vi "novoGoleiroGoleiroForaDaArea.vi"(9 "Goleiro.Xpadrão":dbl=80.0 format="%#_13g", 10 "Robot in":T1, 11 "IA State":T6={"our_robots"=[], "enemy_robots"=[], "balls"=[], "geometry"={"field_length"=0, "field_width"=0, "goal_width"=0, "goal_depth"=0, "center_circle_radius"=0, "defense_width"=0, "defense_depth"=0, "free_kick_from_defense_dist"=0, "penalty_spot_from_field_line_dist"=0, "penalty_line_from_spot_dist"=0, "half_moon_depth"=0, "half_moon_width"=0}, "IA Judge"={"stage"="", "command"="", "our_goalie_id"=0.0, "enemy_goalie_id"=0.0, "command enum"=enum."Halt", "Time"=enum."Azul"}, "Received Timestamp"=timestamp(0 s since 1904-01-01), "Events"={"Touch"=FALSE, "id touch"=0.0, "Ball out of \nVision"=FALSE, "Ball inside \nGoalie area"=FALSE, "Robot not responding"=FALSE, "Robots responding status"=[1.0, 1.0, 1.0, 1.0, 1.0, 1.0], "Enemy Ball \nPossession"=FALSE, "Id ini Possession"=0.0, "Ball Possesion"=FALSE, "Id Possesion"=0.0, "Ball at\nour goal side"=FALSE, "Ball at\ntouchline"=FALSE, "Ball at\nenemy goal side"=FALSE}}) -> (3 "Cluster de saída":T1)   [LabVIEW 2018]
doc: "Função que retorna os parâmetros para o controle da VSS,\ndado que está no estado \"Goleiro fora da área\"."
uses:
  2019/VSS/Core/AI Robot.ctl
  2019/VSS/Intel/Functions Enum.ctl
  2019/VSS/Intel/AttackerStates.ctl
  2019/VSS/Path Planning/RRT/PathDests.ctl
  2019/VSS/Path Planning/RRT/PathDest.ctl
  2019/VSS/Core/AI Input.ctl
  2019/VSS/Core/AI Ball.ctl
  2019/VSS/Core/Field Size.ctl
  2019/VSS/Core/AI Judge.ctl
  2019/VSS/Intel/Command Enum.ctl
  2019/VSS/Util/Events/Events.ctl
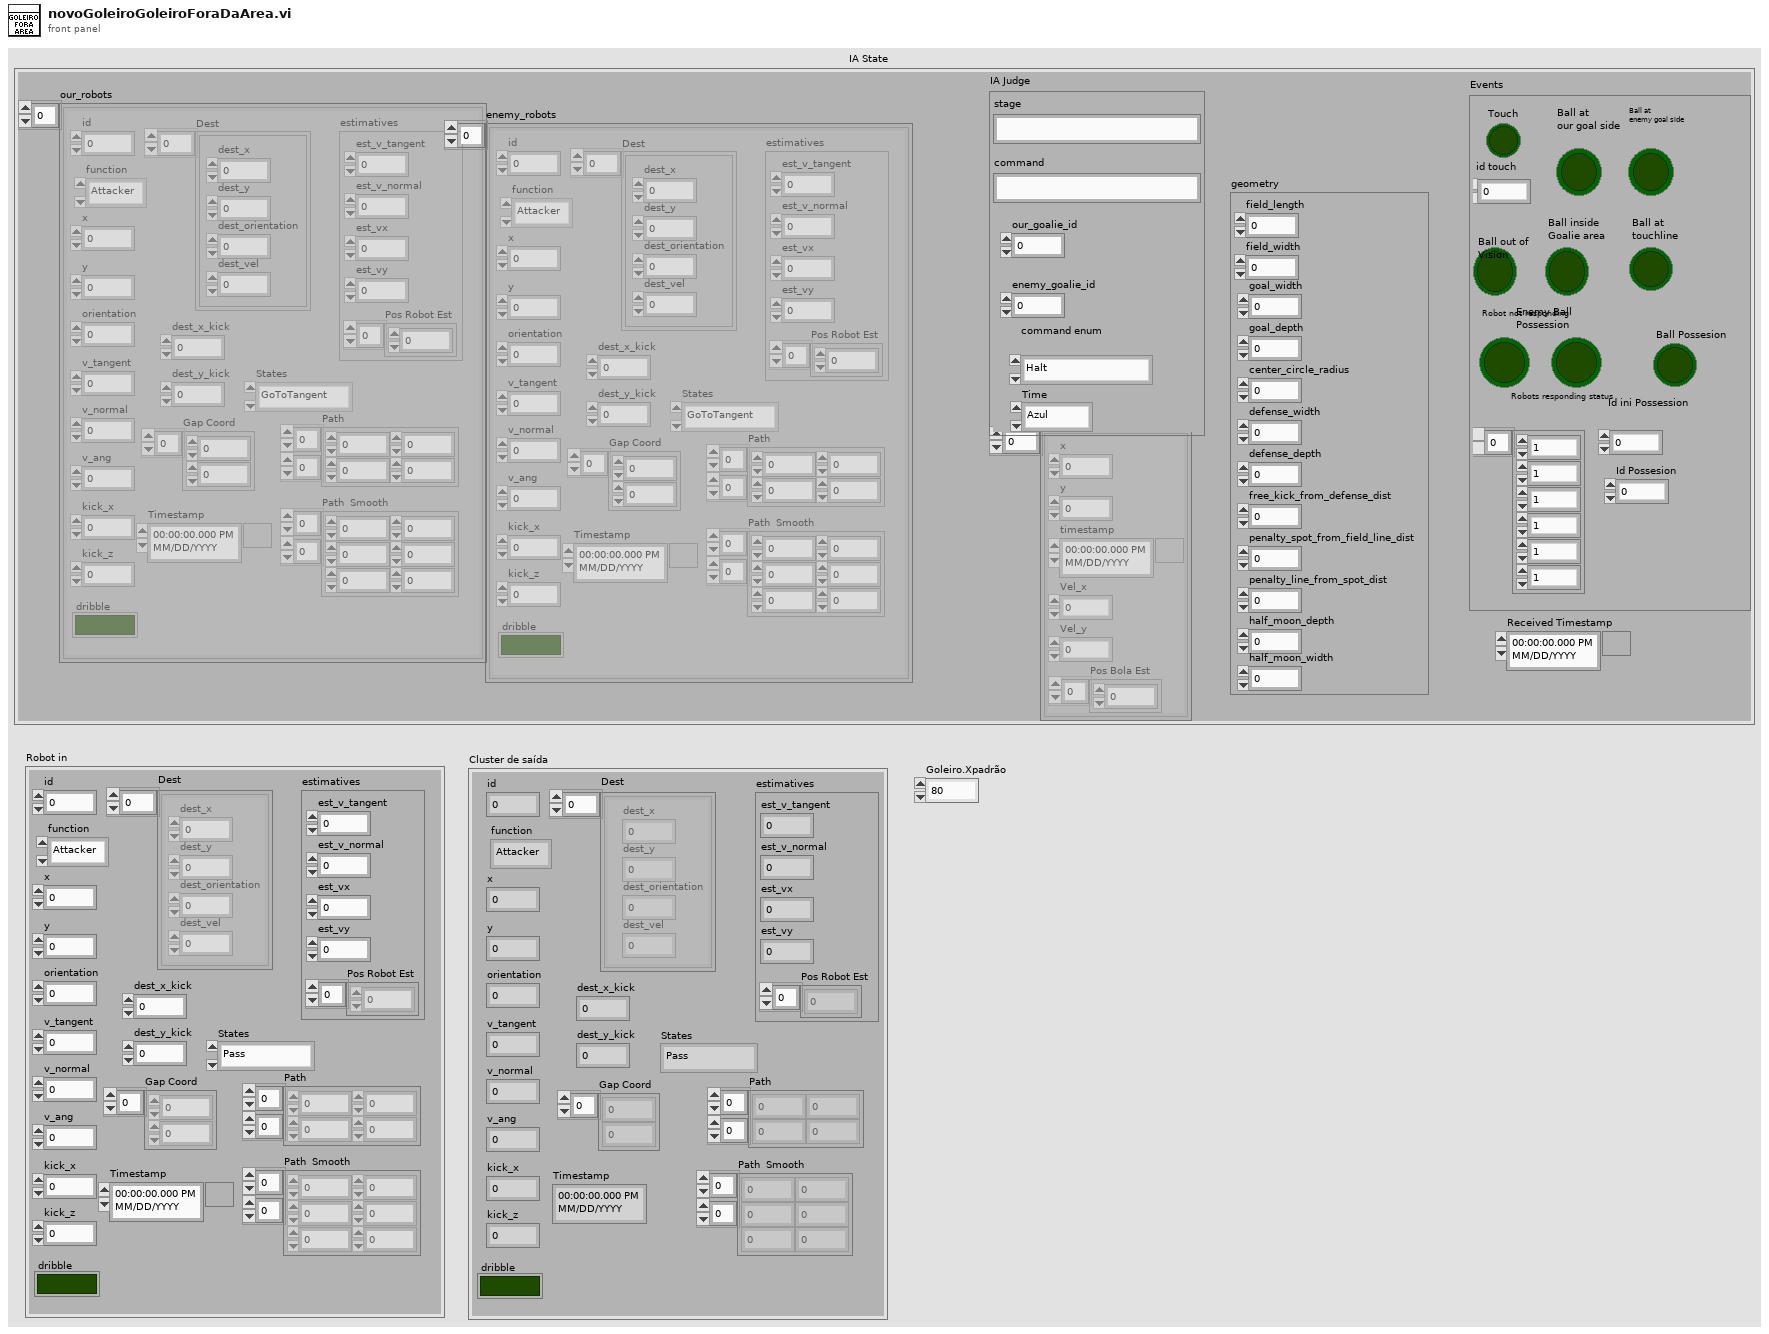
[diagram p1: front panel]
types:
  T1 = typedef "AI Robot.ctl" = cluster{"id":u32, "function":T2, "x":dbl, "y":dbl, "orientation":dbl, "v_tangent":dbl, "v_normal":dbl, "v_ang":dbl, "kick_x":dbl, "kick_z":dbl, "dribble":bool, "Timestamp":timestamp, "estimatives":cluster{"est_v_tangent":dbl, "est_v_normal":dbl, "est_vx":dbl, "est_vy":dbl, "Pos Robot Est":dbl[]}, "dest_x_kick":dbl, "dest_y_kick":dbl, "Gap Coord":dbl[], "States":T3, "Path ":dbl[][], "Path  Smooth":dbl[][], "Dest":T4}
  T2 = typedef "Functions Enum.ctl" = enum16{"Attacker", "Goalie", "Defender", "Striker", "Goto 0", "Dummy", "Kicker", "ZigZag"}
  T3 = typedef "AttackerStates.ctl" = enum16{"Pass", "GoToTangent", "BallGetting", "GoToKick", "Rotate anti-clockwise", "Rotate Clockwise", ""}
  T4 = typedef "PathDests.ctl" = T5[]
  T5 = typedef "PathDest.ctl" = cluster{"dest_x":dbl, "dest_y":dbl, "dest_orientation":dbl, "dest_vel":dbl}
  T6 = typedef "AI Input.ctl" = cluster{"our_robots":T1[], "enemy_robots":T1[], "balls":T7[], "geometry":T8, "IA Judge":T9, "Received Timestamp":timestamp, "Events":T11}
  T7 = typedef "AI Ball.ctl" = cluster{"x":dbl, "y":dbl, "timestamp":timestamp, "Vel_x":dbl, "Vel_y":dbl, "Pos Bola Est":dbl[]}
  T8 = typedef "Field Size.ctl" = cluster{"field_length":u32, "field_width":u32, "goal_width":u32, "goal_depth":u32, "center_circle_radius":u32, "defense_width":u32, "defense_depth":u32, "free_kick_from_defense_dist":u32, "penalty_spot_from_field_line_dist":u32, "penalty_line_from_spot_dist":u32, "half_moon_depth":u32, "half_moon_width":u32}
  T9 = typedef "AI Judge.ctl" = cluster{"stage":string, "command":string, "our_goalie_id":dbl, "enemy_goalie_id":dbl, "command enum":T10, "Time":enum16{"Azul", "Amarelo"}}
  T10 = typedef "Command Enum.ctl" = enum16{"Halt", "Stop", "Force Start", "PKA Normal Start", "Prepare Kickoff Ally", "PKE Normal Start", "Prepare Kickoff Enemy", "Prepare Penalty Ally", "PPA Normal Start", "Prepare Penalty Enemy", "PPE Normal Start", "Ball Placement Enemy Up", "Ball Placement Enemy Down", "Ball Placement Ally Up", "Ball Placement Ally Mid", "Ball Placement Ally Down", "Indirect Free Enemy", "Indirect Free Ally", "Timeout Enemy", "Timeout Ally", "Goal Enemy", "Goal Ally", "Normal Half Time", "Extra Time Break", "Extra Half Time", "None", "Post Game"}
  T11 = typedef "Events.ctl" = cluster{"Touch":bool, "id touch":dbl, "Ball out of \nVision":bool, "Ball inside \nGoalie area":bool, "Robot not responding":bool, "Robots responding status":dbl[], "Enemy Ball \nPossession":bool, "Id ini Possession":dbl, "Ball Possesion":bool, "Id Possesion":dbl, "Ball at\nour goal side":bool, "Ball at\ntouchline":bool, "Ball at\nenemy goal side":bool}
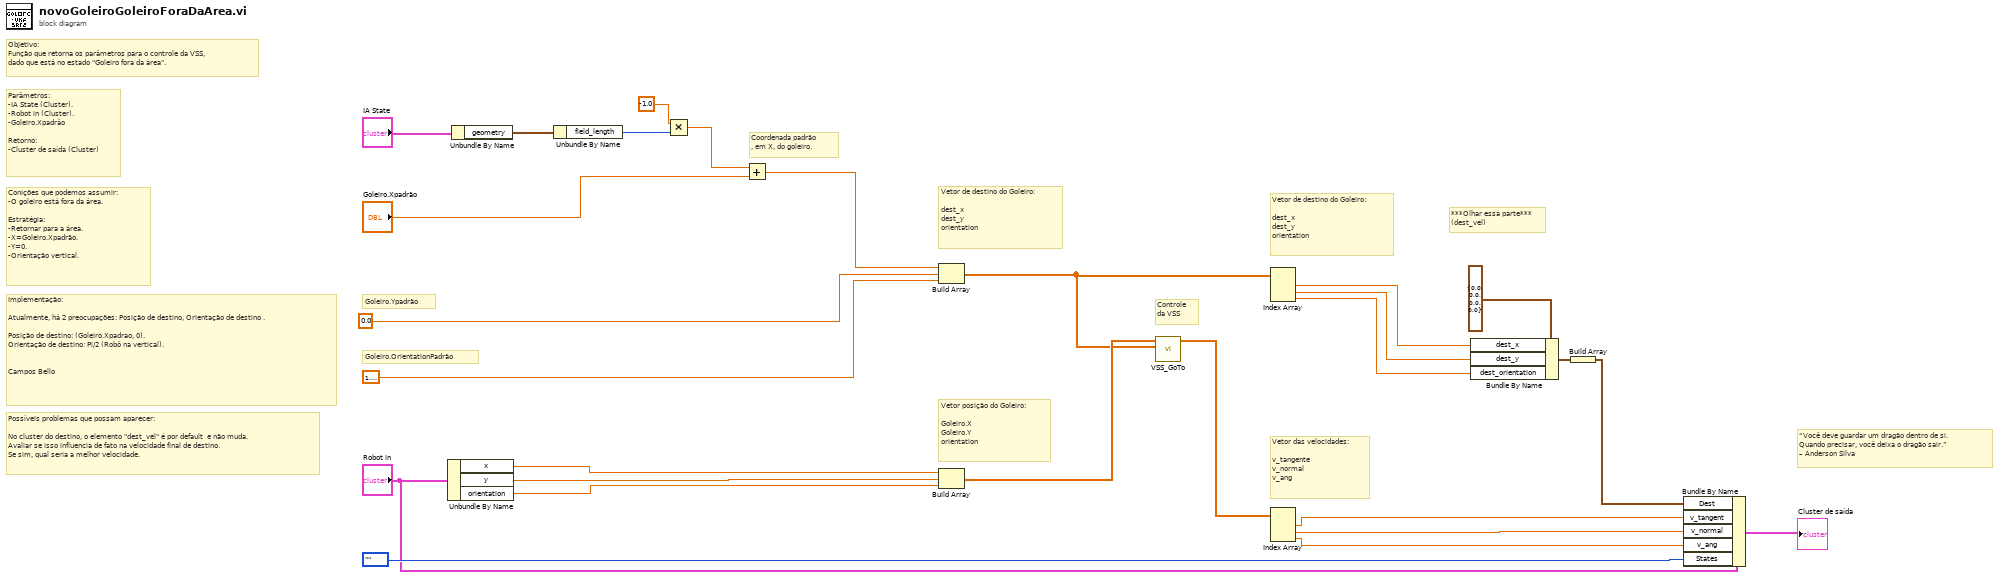
[diagram p0: block diagram]
diagram:
  # "Conições que podemos assumir:\n-O goleiro está fora da área.\n\nEstratégia:\n-Retornar para a área.\n-X=Goleiro.Xpadrão.\n-Y=0.\n-Orientação vertical."
  # "Possíveis problemas que possam aparecer:\n\nNo cluster do destino, o elemento \"dest_vel\" é por default  e não muda. \nAvaliar se isso influencia de fato na velocidade final de destino.\nSe sim, qual seria a melhor velocidade."
  # "Implementação:\n\nAtualmente, há 2 preocupações: Posição de destino, Orientação de destino .\n\nPosição de destino: (Goleiro.Xpadrao, 0).\nOrientação de destino: Pi/2 (Robô na vertical).\n\n\nCampos Bello"
  # "Parâmetros:\n-IA State (Cluster).\n-Robot in (Cluster).\n-Goleiro.Xpadrâo\n\nRetorno:\n-Cluster de saída (Cluster)"
  # "Objetivo:\nFunção que retorna os parâmetros para o controle da VSS,\ndado que está no estado \"Goleiro fora da área\"."
  # "“Você deve guardar um dragão dentro de si. \nQuando precisar, você deixa o dragão sair.” \n– Anderson Silva"
  # "Vetor de destino do Goleiro:\n\ndest_x\ndest_y\norientation"
  # "Vetor das velocidades:\n\nv_tangente\nv_normal\nv_ang"
  # "***Olhar essa parte***\n(dest_vel)"
  # "Vetor posição do Goleiro:\n\nGoleiro.X\nGoleiro.Y\norientation"
  # "Controle \nda VSS"
  # "Vetor de destino do Goleiro:\n\ndest_x\ndest_y\norientation"
  # "Coordenada padrão\n, em X, do goleiro."
  # "Goleiro.OrientationPadrão"
  # "Goleiro.Ypadrão"
  n1 = Unbundle By Name("Robot in") -> ("x"=w16:dbl, "y"=w15:dbl, "orientation"=w14:dbl)
  n2 = Unbundle By Name("IA State") -> ("geometry"=w26:T8)
  n3 = Unbundle By Name(w26) -> ("field_length"=w24:u32)
  n4 = Multiply(x=-1.0 ("x*y"), y=w24) -> (x*y=w22:dbl)
  n5 = Add(x=w22, y="Goleiro.Xpadrão") -> (x+y=w21:dbl)
  n6 = Build Array(w21, 0.0, 1.5707963267948966) -> (w5:dbl[])
  n7 = Build Array(w16, w15, w14) -> (w13:dbl[])
  n8 = call "VSS_GoTo.vi"("SetPoint"=w5, "Position"=w13) -> ("Output Vel"=w9:dbl[])  [unwired: 9 in]
  n9 = Index Array(array=w5) -> (element #1=w4:dbl, element #2=w3:dbl, element #3=w2:dbl)  [unwired: 3 in]
  n10 = Index Array(array=w9) -> (element #1=w8:dbl, element #2=w7:dbl, element #3=w6:dbl)  [unwired: 3 in]
  n11 = Bundle By Name(cluster=T5 {"dest_x"=0.0, "dest_y"=0.0, "dest_orientation"=0.0, "dest_vel"=0.0} ("element"), "dest_x"=w4, "dest_y"=w3, "dest_orientation"=w2) -> (w11:T5)
  n12 = Build Array(w11) -> (w10:T5[])
  n13 = Bundle By Name(cluster="Robot in", "Dest"=w10, "v_tangent"=w8, "v_normal"=w7, "v_ang"=w6, "States"=AttackerStates."") -> (→"Cluster de saída":T1)
